vi "Read ROV String_SIL.vi"(8 "error in (no error)":errorcluster, 9 "NAVI string":string="!init;50;70;0;0;;;;", 10 "ROV string":string="34.5,,,,$56.3,34.556,,,,$67.9", 11 "Vessel in":refnum<class "Vessel.lvclass">) -> (0 "error out":errorcluster, 1 "dvl_m":dbl[](array[numeric]), 2 "Signals out":dbl[](array[numeric]), 3 "Vessel out":refnum<class "Vessel.lvclass">)   [LabVIEW 2014, in "Vessel.lvclass"]
uses:
  Vessel.lvclass
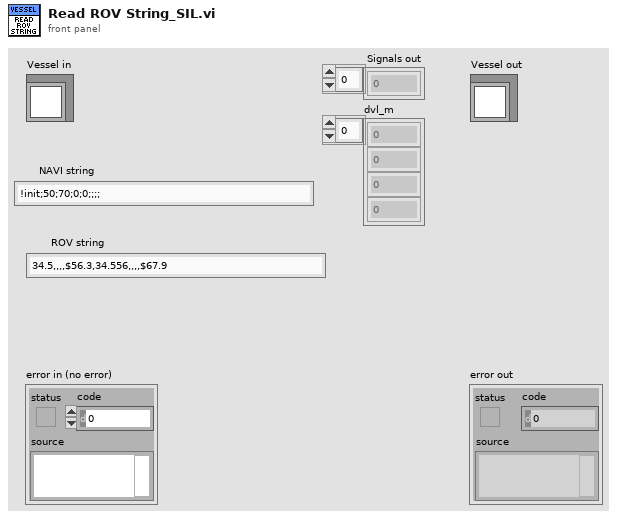
[diagram p1: front panel]
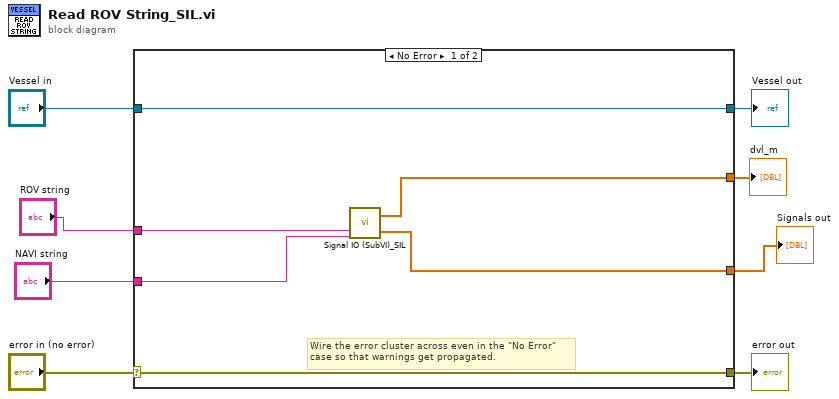
[diagram p0: block diagram]
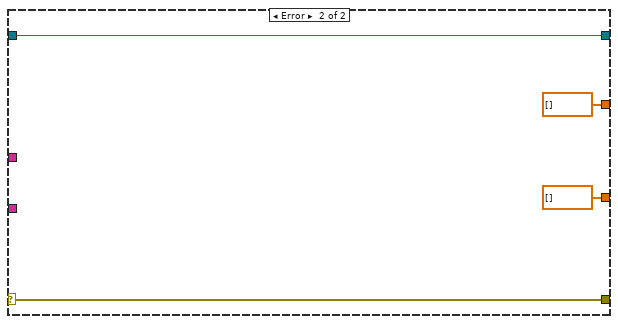
[diagram p2: hidden frame]
diagram:
  n1 = case shown="No Error" "error in (no error)" {
    selector: "error in (no error)" -> [w13 w18]
    tunnel: [w13 w18] -> w7
    tunnel: [w14 w17] -> w5
    tunnel: "Vessel in" -> [w14 w17]
    tunnel: "ROV string" -> [w12 _]
    tunnel: "NAVI string" -> [w11 _]
    tunnel: [w10 dbl[] [] ("Signals out")] -> w2
    tunnel: [w9 dbl[] [] ("dvl_m")] -> w1
    frame No Error {
      # "Wire the error cluster across even in the \"No Error\"\ncase so that warnings get propagated."
      n2 = call "Signal IO (SubVI)_SIL.vi"("ROV string"=w12, "NAVI string"=w11) -> ("dvl_m"=w9:dbl[], "Signals out"=w10:dbl[])  [unwired: 12 in, 4 out]
    }
    frame Error {
    }
  }
  "error out" <- w7
  "Vessel out" <- w5
  "Signals out" <- w2
  "dvl_m" <- w1
